vi "Measure Voltage.vi"(8 "rate":dbl=1000.0 format="%0.2f", 9 "Measure time (s)":dbl=1.0, 11 "physical channels":tag) -> (0 "error out":errorcluster, 1 "RMS":dbl[](array[numeric]), 2 "DC":dbl[](array[numeric]), 3 "Ouput waveform":dbl[][](graph))   [LabVIEW 2012]
uses:
  <vilib>/DAQmx/create/channels.llb/DAQmx Create Channel (AI-Voltage-Basic).vi
  <vilib>/DAQmx/configure/timing.llb/DAQmx Timing (Sample Clock).vi
  <vilib>/measure/NI_MAPro.lvlib
  <vilib>/measure/madcrms.llb/Basic Averaged DC-RMS for 1 Chan.vi
  <vilib>/DAQmx/read.llb/DAQmx Read (Analog 2D DBL NChan NSamp).vi
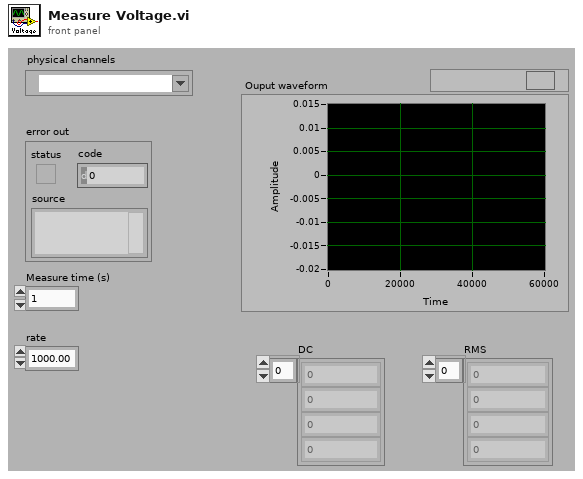
[diagram p1: front panel]
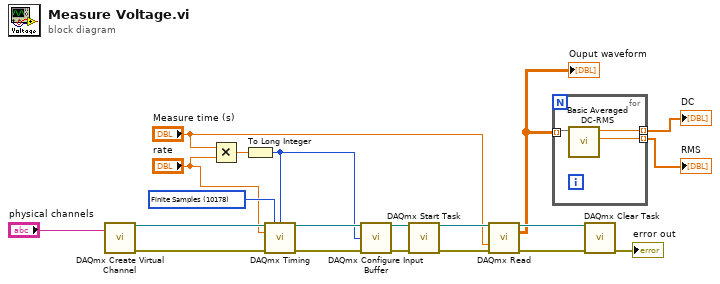
[diagram p0: block diagram]
diagram:
  w20 = 10178 items=["Finite Samples"=10178, "Continuous Samples"=10123, "Hardware Timed Single Point"=12522] ("sample mode")
  n1 = call-poly <vilib>:"DAQmx Create Virtual Channel.vi"("physical channels"="physical channels") -> ("task out"=w19:refnum<k21>, "error out"=w18:errorcluster)  [unwired: 13 in]
  n2 = Multiply(x="Measure time (s)", y="rate") -> (x*y=w11:dbl)
  n3 = To Long Integer(number=w11) -> (32bit integer=w2:i32)
  n4 = call-poly <vilib>:"DAQmx Timing.vi"("task/channels in"=w19, "sample mode"=w20, "samples per channel"=w2, "rate"="rate", "error in"=w18) -> ("task out"=w6:refnum<k21>, "error out"=w4:errorcluster)  [unwired: 9 in]
  n5 = call <vilib>:"DAQmx Configure Input Buffer.vi"("task/channels in"=w6, "buffer size (in samples per channel)"=w2, "error in"=w4) -> ("task out"=w5:refnum<k21>, "error out"=w3:errorcluster)  [unwired: 11 in]
  n6 = call <vilib>:"DAQmx Start Task.vi"("task/channels in"=w5, "error in"=w3) -> ("task out"=w16:refnum<k21>, "error out"=w15:errorcluster)  [unwired: 12 in]
  n7 = call-poly <vilib>:"DAQmx Read.vi"("task/channels in"=w16, "timeout"="Measure time (s)", "error in"=w15) -> ("task out"=w14:refnum<k21>, "data"=w9:dbl[][], "error out"=w13:errorcluster)  [unwired: 10 in]
  "Ouput waveform" <- w9
  n8 = for {
    tunnel: [w23] -> w8 mode=indexing
    tunnel: [w22] -> w7 mode=indexing
    tunnel: w9 -> [w21] mode=indexing
    n9 = call-poly <vilib>:"Basic Averaged DC-RMS.vi"("signal in"=w21) -> ("RMS value"=w22:dbl, "DC value"=w23:dbl)  [unwired: 7 in, 2 out]
  }
  "DC" <- w8
  "RMS" <- w7
  n10 = call <vilib>:"DAQmx Clear Task.vi"("task in"=w14, "error in"=w13) -> ("error out"=→"error out":errorcluster)  [unwired: 13 in]
